vi "Get LIN Schedule Rate.vi"(8 "error in (no error)":errorcluster, 10 "Frame Ref":refnum<k24>, 11 "XNET Cluster":refnum<k21>) -> (0 "error out":errorcluster, 1 "Rate":dbl, 2 "Frame Ref out":refnum<k24>, 3 "XNET Cluster out":refnum<k21>)   [LabVIEW 2015, in "Protection and Rolling Counter Addon System Explorer.lvlib"]
uses:
  Protection and Rolling Counter Addon System Explorer.lvlib
  NationalInstruments.VeriStand.SystemStorage
  <resource>/objmgr/xnet.rc
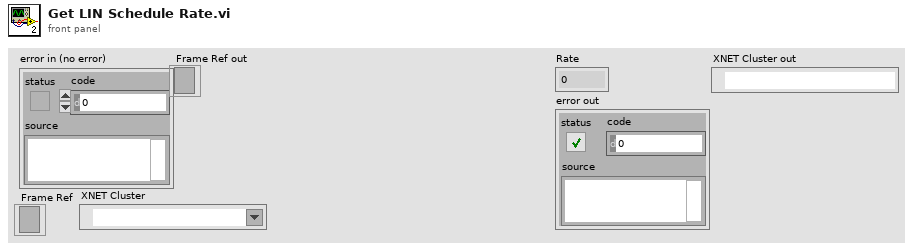
[diagram p1: front panel]
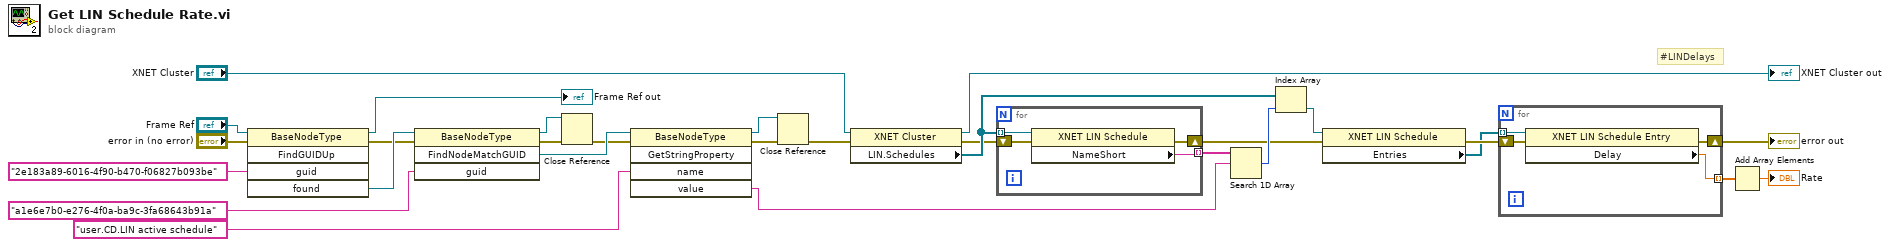
[diagram p0: block diagram]
diagram:
  # "#LINDelays"
  n1 = invoke class="BaseNodeType" method="FindGUIDUp"(reference="Frame Ref", error in="error in (no error)", "guid"="2e183a89-6016-4f90-b470-f06827b093be") -> (reference out=→"Frame Ref out":refnum<k24>, error out=w15:errorcluster, "found"=w17:refnum<k24>)  [unwired: 2 in, 2 out]
  n2 = invoke class="BaseNodeType" method="FindNodeMatchGUID"(reference=w17, error in=w15, "guid"="a1e6e7b0-e276-4f0a-ba9c-3fa68643b91a" ("Property Name")) -> (reference out=w6:refnum<k24>, error out=w12:errorcluster, "FindNodeMatchGUID"=w13:refnum<k24>)  [unwired: 1 in, 1 out]
  n3 = Close Reference(reference=w6, error in (no error)=w12) -> (error out=w7:errorcluster)
  n4 = invoke class="BaseNodeType" method="GetStringProperty"(reference=w13, error in=w7, "name"="user.CD.LIN active schedule" ("Property Name")) -> (reference out=w5:refnum<k24>, error out=w4:errorcluster, "value"=w2:string)  [unwired: 2 in, 2 out]
  n5 = Close Reference(reference=w5, error in (no error)=w4) -> (error out=w3:errorcluster)
  n6 = property class="XNET Cluster"(reference="XNET Cluster", error in=w3) -> (reference out=→"XNET Cluster out":refnum<k21>, error out=w21:errorcluster, "LIN.Schedules"=w25:refnum<k21>[])
  n7 = for {
    tunnel: [w33] -> w24 mode=indexing
    tunnel: w25 -> [w32] mode=indexing
    shift-right: [w30] -> w20
    shift-left: w21 -> [w31]
    n8 = property class="XNET LIN Schedule"(reference=w32, error in=w31) -> (error out=w30:errorcluster, "NameShort"=w33:string)  [unwired: 1 out]
  }
  n9 = Search 1D Array(1D array=w24, element=w2) -> (index of element=w23:i32)  [unwired: 1 in]
  n10 = Index Array(array=w25, index=w23) -> (element=w29:refnum<k21>)
  n11 = property class="XNET LIN Schedule"(reference=w29, error in=w20) -> (error out=w28:errorcluster, "Entries"=w27:refnum<k21>[])  [unwired: 1 out]
  n12 = for {
    tunnel: w27 -> [w34] mode=indexing
    tunnel: [w36] -> w26 mode=indexing
    shift-right: [w35] -> w22
    shift-left: w28 -> [w37]
    n13 = property class="XNET LIN Schedule Entry"(reference=w34, error in=w37) -> (error out=w35:errorcluster, "Delay"=w36:dbl)  [unwired: 1 out]
  }
  "error out" <- w22
  n14 = Add Array Elements(numeric array=w26) -> (sum=→"Rate":dbl)
